vi "Write Creation TS.vi"(8 "error in (no error)":errorcluster, 10 "Start Creation":u64, 11 "CIFCorePlugin in":refnum<class "CIFCorePlugin.lvclass">) -> (0 "error out":errorcluster, 3 "CIFCorePlugin out":refnum<class "CIFCorePlugin.lvclass">)   [LabVIEW 2021, in "CIFCorePlugin.lvclass"]
doc: "Update the timestamp. Time is U64, absolute time in nS in the appropriate clockID configured for the plugin. If a 0 is wired it will automatically get the current time."
uses:
  CIFCorePlugin.lvclass
  CIFCorePlugin.lvclass/CIFCorePlugin.ctl
  Typedef/Log Type.ctl
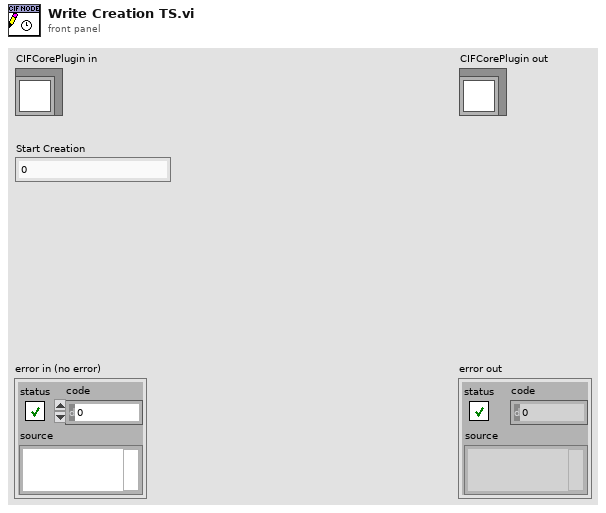
[diagram p1: front panel]
types:
  T1 = typedef "CIFCorePlugin.lvclass/Log Type.ctl" = enum16{"Info", "Config"}
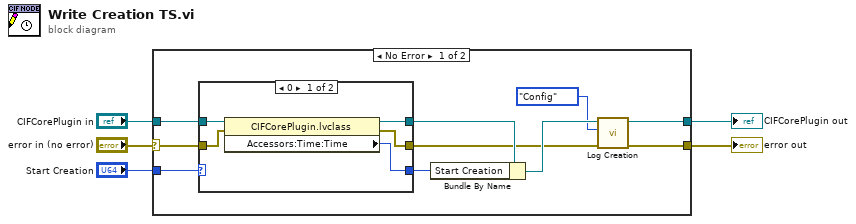
[diagram p0: block diagram]
diagram:
  n1 = case shown="No Error" "error in (no error)" {
    selector: "error in (no error)" -> [w14 w24]
    tunnel: [w7 w24] -> w4
    tunnel: [w8 w25] -> w2
    tunnel: "CIFCorePlugin in" -> [w13 w25]
    tunnel: "Start Creation" -> [w15 _]
    frame No Error {
      n2 = case shown="0" w15 {
        selector: w15 -> [_ w22]
        tunnel: w14 -> [w17 w21]
        tunnel: w13 -> [w20 w23]
        tunnel: [w19 w23] -> w12
        tunnel: [w18 w22] -> w11
        tunnel: [w16 w21] -> w9
        frame 0 {
          n3 = property class="CIFCorePlugin.lvclass"(reference=w20, error in=w17) -> (reference out=w19:refnum<class "CIFCorePlugin.lvclass">, error out=w16:errorcluster, "Accessors:Time:Time"=w18:u64)
        }
        frame 1, Default {
        }
      }
      n4 = Bundle By Name(cluster=w12, "Start Creation"=w11) -> (w10:refnum<class "CIFCorePlugin.lvclass">)
      n5 = call "Log Creation.vi"("error in (no error)"=w9, "Log Type"=Log_Type."Config", "CIFCorePlugin in"=w10) -> ("error out"=w7:errorcluster, "CIFCorePlugin out"=w8:refnum<class "CIFCorePlugin.lvclass">)  [unwired: 7 in]
    }
    frame Error {
    }
  }
  "error out" <- w4
  "CIFCorePlugin out" <- w2
